vi "Create LVObjectArrayMsg.vi"(8 "error in (no error)":errorcluster, 10 "Message Data":refnum<class>[](array[class]), 11 "Message Name":string) -> (0 "error out":errorcluster, 3 "LVObjectArrayMsg out":refnum<class "LVObjectArrayMsg.lvclass">)   [LabVIEW 2013, in "LapDog.Messaging.v3.NativeArrays.lvlib" / "LVObjectArrayMsg.lvclass"]
doc: "Returns a LVObjectArrayMsg object with the given name.\n\nThis method executes regardless of the error in state."
uses:
  LVObjectArrayMsg.lvclass
  LapDog.Messaging/Message/Message.lvclass
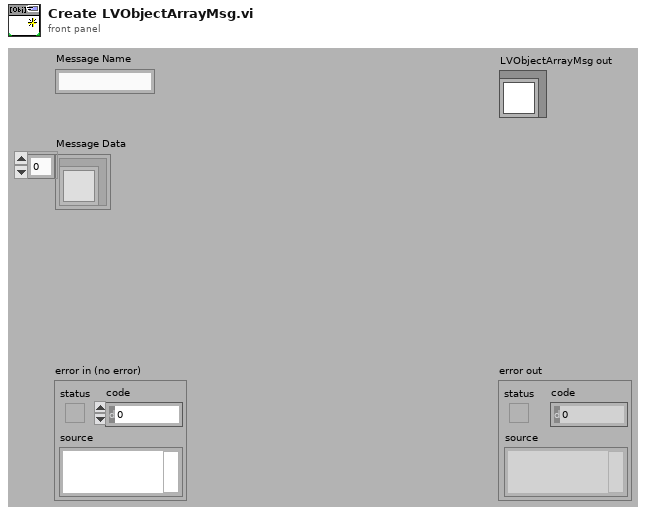
[diagram p1: front panel]
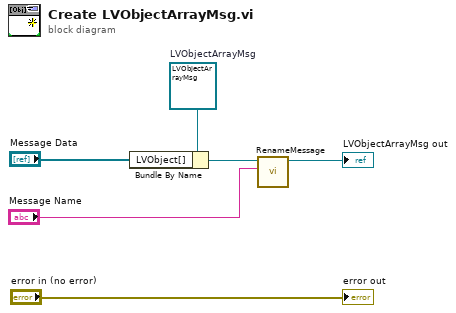
[diagram p0: block diagram]
diagram:
  w1 = refnum<class "LVObjectArrayMsg.lvclass"> refnum  # LVObjectArrayMsg
  n1 = Bundle By Name(cluster=w1, "LVObject[]"="Message Data") -> (w4:refnum<class "LVObjectArrayMsg.lvclass">)
  n2 = call "RenameMessage.vi"("Message Name"="Message Name", "Message in"=w4) -> ("Message out"=→"LVObjectArrayMsg out":refnum<class "LVObjectArrayMsg.lvclass">)  [unwired: 8 in, 1 out]
  "error out" <- "error in (no error)"
